vi "CD_MGR Run.vi"(8 "error in (no error)":errorcluster, 9 "Lasers ON?":bool, 10 "data value reference":refnum<data-value>, 11 "Move Length":i32) -> (0 "error out":errorcluster, 1 "timed out?":bool, 2 "Start Collect (Reply Payload)":T1)   [LabVIEW 2015, in "Collect Data Mgr.lvlib"]
uses:
  Collect Data Mgr.lvlib
  Start Collect (Reply Payload)--cluster.ctl
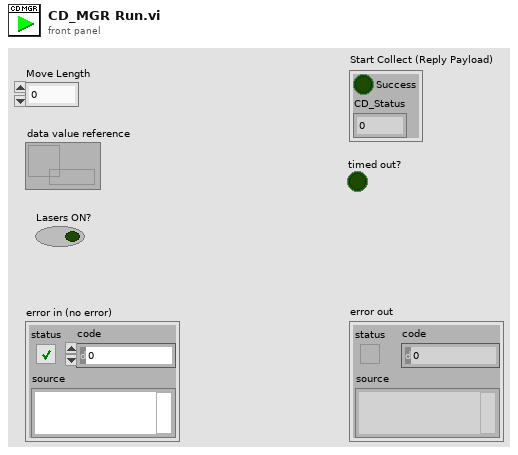
[diagram p1: front panel]
types:
  T1 = typedef "Collect Data Mgr.lvlib/Start Collect (Reply Payload)--cluster.ctl" = cluster{"Success":bool, "CD_Status":u8}
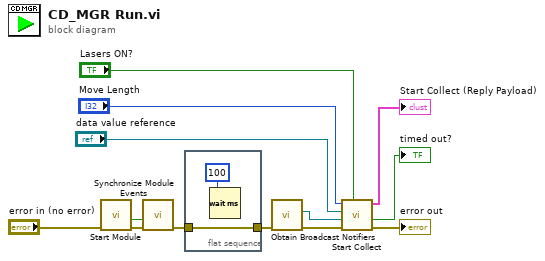
[diagram p0: block diagram]
diagram:
  n1 = call "Start Module.vi"("error in (no error)"="error in (no error)") -> ("error out"=w12:errorcluster, "Wait for Event Sync?"=w13:bool)  [unwired: 8 in, 1 out]
  n2 = call "Synchronize Module Events.vi"("error in (no error)"=w12, "Wait for Event Sync?"=w13) -> ("error out"=w3:errorcluster)  [unwired: 9 in]
  n3 = flat-sequence {
    tunnel: w3 -> [w14]
    tunnel: [w14] -> w2
    frame #0 {
      n4 = Wait (ms)(milliseconds to wait=u32 100) -> ()  [unwired: 1 out]
    }
  }
  n5 = call "Obtain Broadcast Notifiers.vi"("error in (no error)"=w2) -> ("error out"=w7:errorcluster, "Sample Data notifier out"=w6:refnum<notifier>)  [unwired: 9 in]
  n6 = call "Start Collect.vi"("Lasers ON?"="Lasers ON?", "error in (no error)"=w7, "Sample Data notifier"=w6, "data value reference"="data value reference", "Move Length"="Move Length") -> ("error out"=→"error out":errorcluster, "timed out?"=→"timed out?":bool, "Start Collect (Reply Payload)"=→"Start Collect (Reply Payload)":T1)  [unwired: 4 in]
